vi "VG_ATEQ.vi"() -> ()   [LabVIEW 2020]
panel:
  in  "ATEQ":string
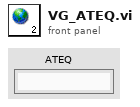
[diagram p1: front panel]
diagram:
